vi "NET DumpToPbtxt.vi"(8 "error in (no error)":errorcluster, 10 "Path":path, 11 "NET in":refnum<class "NET.lvclass">) -> (0 "error out":errorcluster, 3 "NET out":refnum<class "NET.lvclass">)   [LabVIEW 2020, in "OpenLvVision_OpenCv.lvlib" / "NET.lvclass"]
doc: "Dump net structure, hyperparameters, backend, target and fusion to pbtxt file. \nUse Netron (https://netron.app) to open the target file to visualize the model. Call method after setInput(). To see correct backend, target and fusion run after forward()."
uses:
  NET.lvclass
  OpenLvVision_OpenCv.lvlib
  _LvHelpers/EdvrObject/EdvrObject.lvclass
  C:/Users/lukas/Downloads/OpenLvVision_OpenCv/SourceCode/LabView/OpenLvVision_OpenCv/_LvHelpers/EdvrObject/EdvrObject.lvclass
  Dlls/OlvOpenCvWrapper.dll
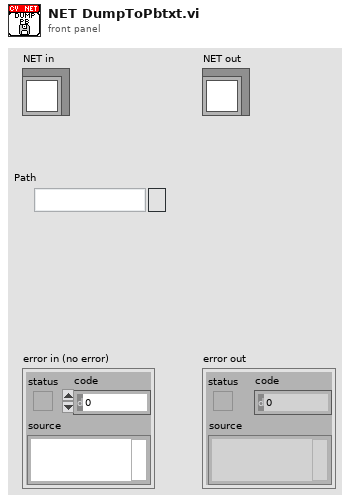
[diagram p1: front panel]
types:
  T1 = typedef "OpenLvVision_OpenCv.lvlib/EdvrObject.lvclass/Edvr.ctl" = refnum<data-value>
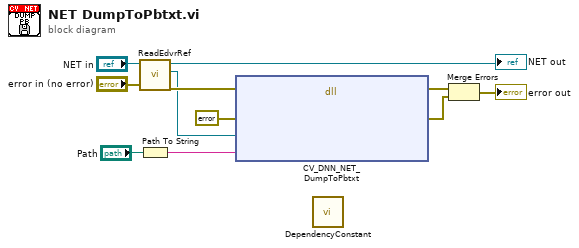
[diagram p0: block diagram]
diagram:
  n1 = call "ReadEdvrRef.vi"("error in (no error)"="error in (no error)", "EdvrObject in"="NET in") -> ("error out"=w7:errorcluster, "Edvr"=w6:T1, "EdvrObject out"=→"NET out":refnum<class "NET.lvclass">)  [unwired: 7 in]
  n2 = Path To String(path="Path") -> (string=w1:string)
  n3 = dll-call lib="C:/Users/lukas/Downloads/OpenLvVision_OpenCv/SourceCode/LabView/OpenLvVision_OpenCv/Dlls/OlvOpenCvWrapper.dll" fn="CV_DNN_NET_DumpToPbtxt"(error in=w7, "Error"=errorcluster {"status"=FALSE, "code"=0, "source"=""} ("error out"), "edvrRef"=w6, "path"=w1) -> (error out=w10:errorcluster, "Error"=w3:errorcluster)  [unwired: 5 in, 1 out]
  n4 = call "DependencyConstant.vi"() -> ()  [unwired: 12 in]
  n5 = Merge Errors(w10, w3) -> (→"error out":errorcluster)
